vi "SimpleMotorTestGUI.vi"() -> ()   [LabVIEW 2009]
uses:
  <vilib>/userDefined/High Color/nirio_resource_hc.ctl
  <vilib>/rvi/interface/nirviOpenFPGA/nirviOpenFPGA.xnode
  Brian Brain.lvproj_FPGA Target 2_SuperSimpleMotorTe~69.lvbitx
  <vilib>/FPGAPlugInAG/sbRIO-9642/nirviIntfOpen_sbRIO-9642.vi
  <vilib>/rvi/interface/nirviReadWriteControl/nirviReadWriteControl.xnode
  <vilib>/Utility/error.llb/Error Cluster From Error Code.vi
  <vilib>/rvi/errors/niLvFpgaAdjustHostInterfaceError.vi
  <vilib>/rvi/interface/common/niFpgaNodeNameForErrorReporting.ctl
  <vilib>/rvi/errors/niLvFpgaWhatHappensToTopLevelVI.ctl
  NiRioSrv.dll
panel:
  in  "resource name":T1
  in  "stop":bool
  in  "M2 Enable":bool
  in  "M1 Enable":bool
  in  "M0 Enable":bool
  in  "M2 output":fxp<+/-,20,5> format="%.17g"
  in  "M1 output":fxp<+/-,20,5> format="%.17g"
  in  "M0 output":fxp<+/-,20,5> format="%.17g"
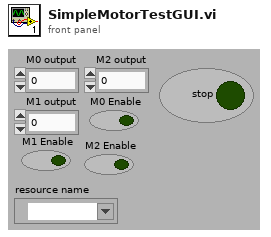
[diagram p1: front panel]
types:
  T1 = typedef "nirio_resource_hc.ctl" = tag
  T2 = typedef "niFpgaNodeNameForErrorReporting.ctl" = enum16{"Open FPGA VI Reference", "Read/Write Control", "Invoke Method: Abort", "Invoke Method: Acknowledge IRQ", "Invoke Method: Download", "Invoke Method: FIFO.Configure", "Invoke Method: FIFO.Read", "Invoke Method: FIFO.Start", "Invoke Method: FIFO.Stop", "Invoke Method: FIFO.Write", "Invoke Method: Reset", "Invoke Method: Run", "Invoke Method: Wait on IRQ", "Close FPGA VI Reference"}
  T3 = typedef "niLvFpgaWhatHappensToTopLevelVI.ctl" = enum16{"top level VI scripted behind XNode", "top level VI inlined behind XNode"}
  T4 = cluster{"signature":u8[], "vi signatures match":bool, "signature register address":u32, "reset register address":u32, "control register address":u32, "interrupt base address":u32, "Bitstream Version":u32, "DMA Configuration":cluster{"Name":string, "Depth":u32, "Write? (Deprecated:Use Implementation)":bool, "Physical Channel":u32, "Base Address":u32, "Data Width":u32, "Data Type":enum32{"Boolean", "I8", "I16", "I32", "I64", "U8", "U16", "U32", "U64", "FXP"}, "FXP Properties":variant, "Write Window Address":u32, "Implementation":enum16{"niFpgaTargetToHost", "niFpgaHostToTarget", "niFpgaPeerToPeerWriter", "niFpgaPeerToPeerReader", "niCoreTargetToHost", "niCoreHostToTarget"}, "Control Set":u32}[], "run when loaded?":bool, "reset register size in bits":u32, "compilation results xml":string}
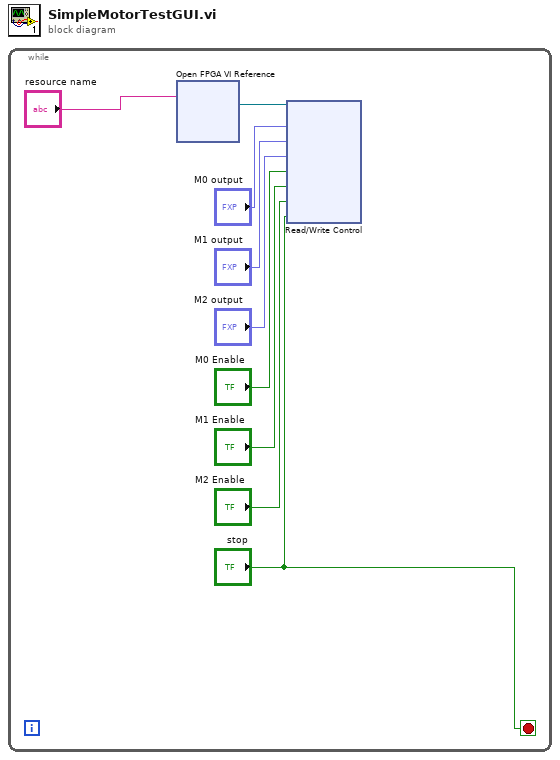
[diagram p0: block diagram]
diagram:
  n1 = while {
    stop <- "stop" stop-if-true
    n2 = xnode "Open FPGA VI Reference"("resource name"="resource name") -> ("FPGA VI Reference Out"=w9:refnum<k20>)  [unwired: 1 in, 1 out]
    n3 = xnode "Read/Write Control"("FPGA VI Reference In"=w9, "M0 output"="M0 output", "M1 output"="M1 output", "M2 output"="M2 output", "M0 Enable"="M0 Enable", "M1 Enable"="M1 Enable", "M2 Enable"="M2 Enable", "stop"="stop") -> ()  [unwired: 1 in, 2 out]
  }
